vi "파일 I_O 실습.vi"() -> ()   [LabVIEW 2020]
uses:
  <vilib>/Utility/sysdir.llb/System Directory Type.ctl
  <vilib>/Utility/file.llb/Read Delimited Spreadsheet (DBL).vi
panel:
  out "연결된 문자열":string
  out "all rows":dbl[][](array[numeric]) caption="모든 행"
  out "데이터 2":string[][](array[string])
  out "데이터":dbl[](array[numeric])
  out "추가된 경로":path
  out "system directory":path caption="시스템 디렉토리"
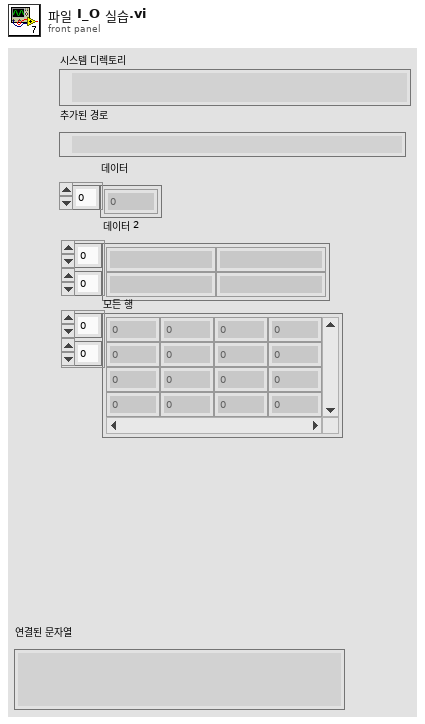
[diagram p1: front panel]
types:
  T1 = enum16{"open", "replace", "create", "open or create", "replace or create", "replace or create with confirmation"}
  T2 = typedef "System Directory Type.ctl" = i32
  T3 = enum16{"open", "open or create", "create or replace", "create", "open (read-only)"}
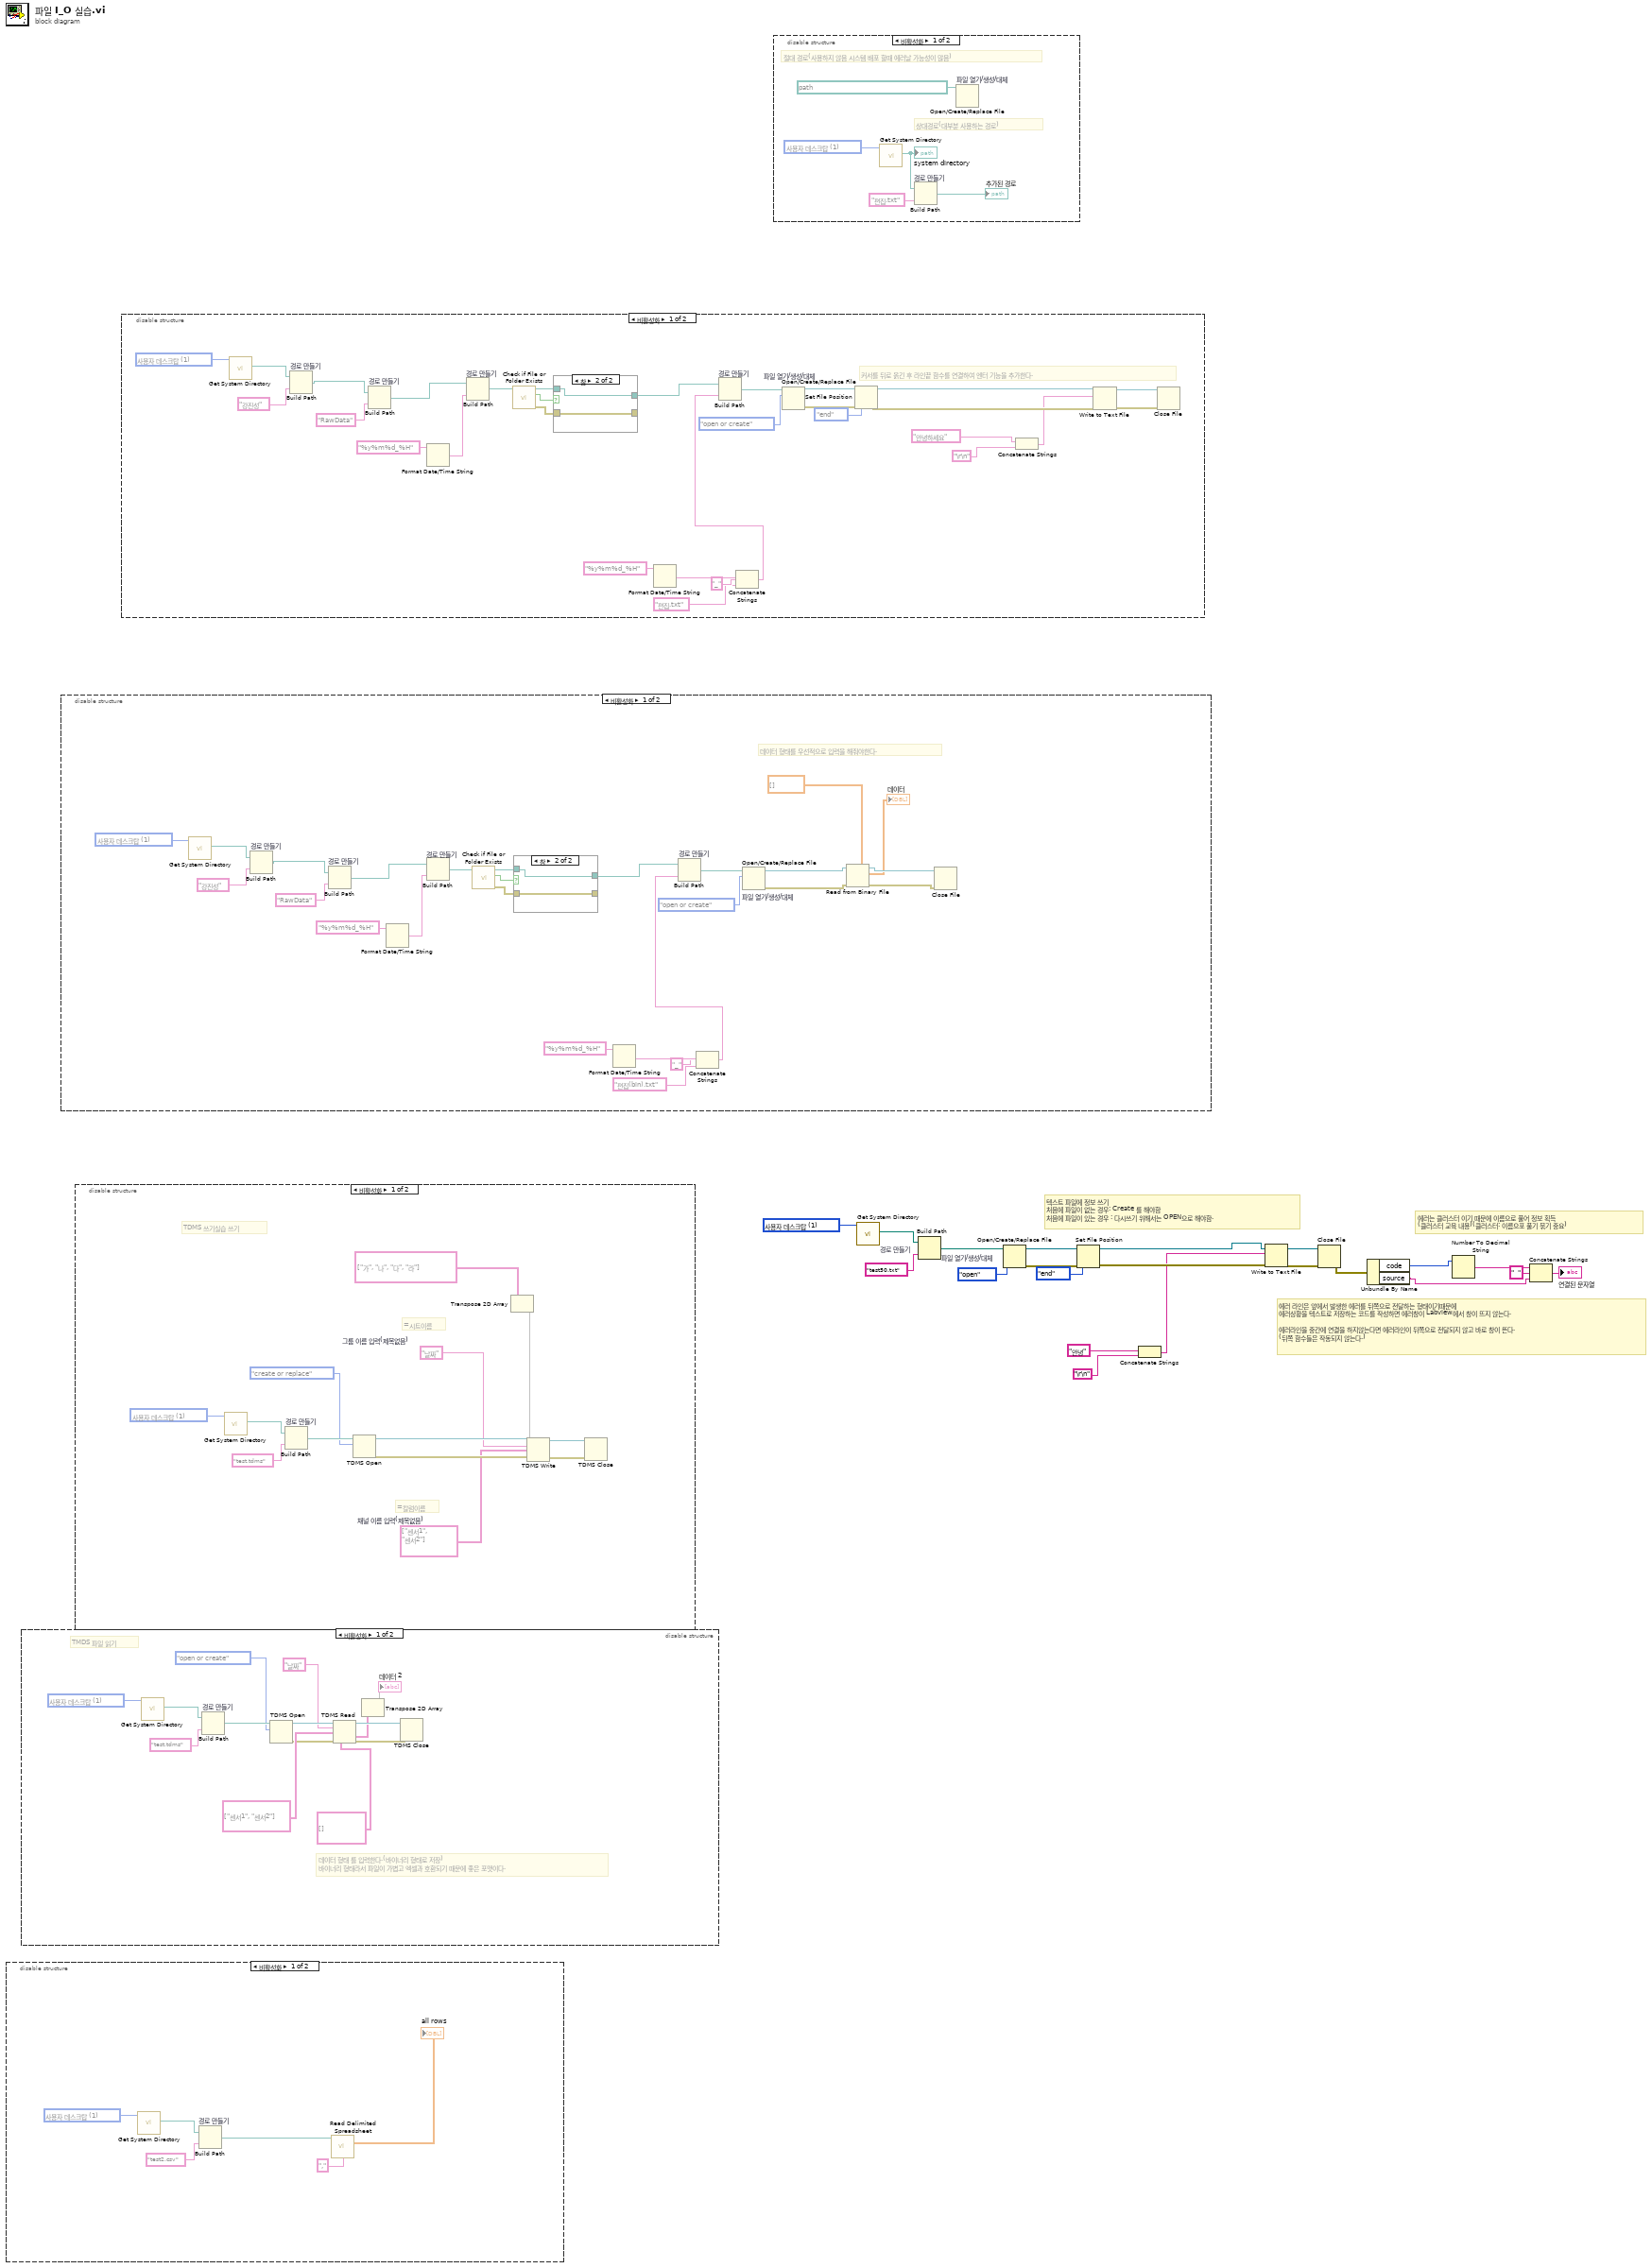
[diagram p0: block diagram]
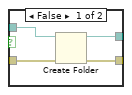
[diagram p5: hidden frame]
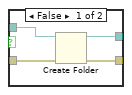
[diagram p7: hidden frame]
diagram:
  w21 = T2 1 items=["사용자 홈"=0, "사용자 데스크탑"=1, "사용자 문서"=2, "사용자 어플리케이션 데이터"=3, "사용자 환경"=4, "사용자 임시"=5, "퍼블릭 문서"=6, "퍼블릭 어플리케이션 데이터"=7, "퍼블릭 환경"=8, "퍼블릭 캐시"=13, "시스템 코어 라이브러리"=9, "시스템 설치된 라이브러리"=10, "어플리케이션 파일"=11, "부팅 볼륨 루트"=12] ("system directory type")
  # "에러 라인은 앞에서 발생한 에러를 뒤쪽으로 전달하는 형태이기때문에\n에러상황을 텍스트로 저장하는 코드를 작성하면 에러창이 Labview에서 창이 뜨지 않는다.\n\n에러라인을 중간에 연결을 하지않는다면 에러라인이 뒤쪽으로 전달되지 않고 바로 창이 뜬다.\n(뒤쪽 함수들은 작동되지 않는다.)"
  # "에러는 클러스터 이기 때문에 이름으로 풀어 정보 획득\n(클러스터 교육 내용)(클러스터: 이름으포 풀기 묶기 중요)"
  # "텍스트 파일에 정보 쓰기\n처음에 파일이 없는 경우: Create 를 해야함\n처음에 파일이 있는 경우 : 다시쓰기 위해서는 OPEN으로 해야함."
  n1 = disable-structure shown="비활성화" {
    frame Disabled {
      w27 = T2 1 items=["사용자 홈"=0, "사용자 데스크탑"=1, "사용자 문서"=2, "사용자 어플리케이션 데이터"=3, "사용자 환경"=4, "사용자 임시"=5, "퍼블릭 문서"=6, "퍼블릭 어플리케이션 데이터"=7, "퍼블릭 환경"=8, "퍼블릭 캐시"=13, "시스템 코어 라이브러리"=9, "시스템 설치된 라이브러리"=10, "어플리케이션 파일"=11, "부팅 볼륨 루트"=12] ("system directory type")
      n2 = call <vilib>:"Get System Directory.vi"("system directory type"=w27) -> ("system directory"=w26:path)  [unwired: 10 in]
      n3 = Build Path "경로 만들기"(base path=w26, name or relative path="test2.csv") -> (appended path=w24:path)
      n4 = call-poly <vilib>:"Read Delimited Spreadsheet.vi"("file path (dialog if empty)"=w24, "delimiter (\\t)"="," ("delimiter (\\t)")) -> ("all rows"=→"all rows":dbl[][])  [unwired: 8 in, 5 out]
    }
    frame Enabled {
    }
  }
  n5 = disable-structure shown="비활성화" {
    frame Disabled {
      w41 = T2 1 items=["사용자 홈"=0, "사용자 데스크탑"=1, "사용자 문서"=2, "사용자 어플리케이션 데이터"=3, "사용자 환경"=4, "사용자 임시"=5, "퍼블릭 문서"=6, "퍼블릭 어플리케이션 데이터"=7, "퍼블릭 환경"=8, "퍼블릭 캐시"=13, "시스템 코어 라이브러리"=9, "시스템 설치된 라이브러리"=10, "어플리케이션 파일"=11, "부팅 볼륨 루트"=12] ("system directory type")
      # "데이터 형태 를 입력한다.(바이너리 형태로 저장)\n바이너리 형태라서 파일이 가볍고 엑셀과 호환되기 때문에 좋은 포맷이다."
      # "TMDS 파일 읽기"
      n6 = call <vilib>:"Get System Directory.vi"("system directory type"=w41) -> ("system directory"=w40:path)  [unwired: 10 in]
      n7 = Build Path "경로 만들기"(base path=w40, name or relative path="test.tdms") -> (appended path=w38:path)
      n8 = TDMS Open(10:T3."open or create" ("동작(0:open)"), 11:w38) -> (0:w31:errorcluster, 3:w36:refnum<k34>)  [unwired: 5 in]
      n9 = TDMS Read(0:w36, 5:"날짜" ("그룹 이름 입력"), 7:string[] ["센서1", "센서2"] ("채널 이름 입력"), 11:w31, 12:string[][] []) -> (4:w33:refnum<k34>, 10:w29:string[][], 15:w32:errorcluster)  [unwired: 3 in, 3 out]
      n10 = Transpose 2D Array(2D array=w29) -> (transposed array=→"데이터 2":string[][])
      n11 = TDMS Close(8:w32, 11:w33) -> ()  [unwired: 2 out]
    }
    frame Enabled {
    }
  }
  n12 = disable-structure shown="비활성화" {
    frame Disabled {
      w67 = T2 1 items=["사용자 홈"=0, "사용자 데스크탑"=1, "사용자 문서"=2, "사용자 어플리케이션 데이터"=3, "사용자 환경"=4, "사용자 임시"=5, "퍼블릭 문서"=6, "퍼블릭 어플리케이션 데이터"=7, "퍼블릭 환경"=8, "퍼블릭 캐시"=13, "시스템 코어 라이브러리"=9, "시스템 설치된 라이브러리"=10, "어플리케이션 파일"=11, "부팅 볼륨 루트"=12] ("system directory type")
      # "데이터 형태를 우선적으로 입력을 해줘야한다."
      n13 = call <vilib>:"Get System Directory.vi"("system directory type"=w67) -> ("system directory"=w64:path)  [unwired: 10 in]
      n14 = Build Path "경로 만들기"(base path=w64, name or relative path="강진성") -> (appended path=w59:path)
      n15 = Build Path "경로 만들기"(base path=w59, name or relative path="RawData") -> (appended path=w58:path)
      n16 = Format Date/Time String(time format string (%c)="%y%m%d_%H" ("시간 포맷 문자열 (%c)")) -> (date/time string=w61:string)  [unwired: 2 in]
      n17 = Build Path "경로 만들기"(base path=w58, name or relative path=w61) -> (appended path=w52:path)
      n18 = call <vilib>:"Check if File or Folder Exists.vi"("path"=w52) -> ("error out"=w49:errorcluster, "file or folder exists?"=w51:bool, "dup path"=w50:path)  [unwired: 8 in]
      n19 = case shown="참" w51 {
        tunnel: w50 -> [w71 w73]
        tunnel: w49 -> [w70 w72]
        tunnel: [w69 w73] -> w48
        tunnel: [w68 w72] -> _
        frame False {
          n20 = Create Folder(path (use dialog)=w71, error in=w70) -> (created path=w69:path, error out=w68:errorcluster)  [unwired: 1 in, 1 out]
        }
        frame True {
        }
      }
      n21 = Format Date/Time String(time format string (%c)="%y%m%d_%H" ("시간 포맷 문자열 (%c)")) -> (date/time string=w56:string)  [unwired: 2 in]
      n22 = Concatenate Strings(w56, "_" ("문자열"), "편집(bin).txt") -> (w53:string)
      n23 = Build Path "경로 만들기"(base path=w48, name or relative path=w53) -> (appended path=w66:path)
      n24 = Open/Create/Replace File "파일 열기/생성/대체"(file path (use dialog)=w66, operation (0:open)=T1."open or create" ("동작(0:open)")) -> (refnum out=w47:refnum<file>, error out=w46:errorcluster)  [unwired: 4 in, 1 out]
      n25 = Read from Binary File(5:dbl[] [], 8:w46, 11:w47) -> (0:w44:errorcluster, 2:→"데이터":dbl[], 3:w45:refnum<file>)  [unwired: 3 in, 1 out]
      n26 = Close File(refnum=w45, error in=w44) -> ()  [unwired: 2 out]
    }
    frame Enabled {
    }
  }
  n27 = disable-structure shown="비활성화" {
    frame Disabled {
      w75 = string[] ["센서1", "센서2"]  # 채널 이름 입력(제목없음)
      w76 = "날짜"  # 그룹 이름 입력(제목없음)
      w86 = T2 1 items=["사용자 홈"=0, "사용자 데스크탑"=1, "사용자 문서"=2, "사용자 어플리케이션 데이터"=3, "사용자 환경"=4, "사용자 임시"=5, "퍼블릭 문서"=6, "퍼블릭 어플리케이션 데이터"=7, "퍼블릭 환경"=8, "퍼블릭 캐시"=13, "시스템 코어 라이브러리"=9, "시스템 설치된 라이브러리"=10, "어플리케이션 파일"=11, "부팅 볼륨 루트"=12] ("system directory type")
      # "TDMS 쓰기실습 쓰기"
      # "=칼럼이름"
      # "=시트이름"
      n28 = call <vilib>:"Get System Directory.vi"("system directory type"=w86) -> ("system directory"=w85:path)  [unwired: 10 in]
      n29 = Build Path "경로 만들기"(base path=w85, name or relative path="test.tdms") -> (appended path=w83:path)
      n30 = TDMS Open(10:T3."create or replace" ("동작(0:open)"), 11:w83) -> (0:w81:errorcluster, 3:w82:refnum<k34>)  [unwired: 5 in]
      n31 = Transpose 2D Array(2D array=string[][] [["가", "나"], ["다", "라"]]) -> (transposed array=w74:string[][])
      n32 = TDMS Write(0:w82, 5:w76, 7:w75, 9:w74, 11:w81) -> (4:w80:refnum<k34>, 15:w79:errorcluster)  [unwired: 1 in, 2 out]
      n33 = TDMS Close(8:w79, 11:w80) -> ()  [unwired: 2 out]
    }
    frame Enabled {
    }
  }
  n34 = disable-structure shown="비활성화" {
    frame Disabled {
      w116 = T2 1 items=["사용자 홈"=0, "사용자 데스크탑"=1, "사용자 문서"=2, "사용자 어플리케이션 데이터"=3, "사용자 환경"=4, "사용자 임시"=5, "퍼블릭 문서"=6, "퍼블릭 어플리케이션 데이터"=7, "퍼블릭 환경"=8, "퍼블릭 캐시"=13, "시스템 코어 라이브러리"=9, "시스템 설치된 라이브러리"=10, "어플리케이션 파일"=11, "부팅 볼륨 루트"=12] ("system directory type")
      # "커서를 뒤로 옭긴 후 라인끝 함수를 연결하여 엔터 기능을 추가한다."
      n35 = call <vilib>:"Get System Directory.vi"("system directory type"=w116) -> ("system directory"=w113:path)  [unwired: 10 in]
      n36 = Build Path "경로 만들기"(base path=w113, name or relative path="강진성") -> (appended path=w108:path)
      n37 = Build Path "경로 만들기"(base path=w108, name or relative path="RawData") -> (appended path=w107:path)
      n38 = Format Date/Time String(time format string (%c)="%y%m%d_%H" ("시간 포맷 문자열 (%c)")) -> (date/time string=w110:string)  [unwired: 2 in]
      n39 = Build Path "경로 만들기"(base path=w107, name or relative path=w110) -> (appended path=w101:path)
      n40 = call <vilib>:"Check if File or Folder Exists.vi"("path"=w101) -> ("error out"=w98:errorcluster, "file or folder exists?"=w100:bool, "dup path"=w99:path)  [unwired: 8 in]
      n41 = case shown="참" w100 {
        tunnel: w99 -> [w120 w122]
        tunnel: w98 -> [w119 w121]
        tunnel: [w118 w122] -> w97
        tunnel: [w117 w121] -> _
        frame False {
          n42 = Create Folder(path (use dialog)=w120, error in=w119) -> (created path=w118:path, error out=w117:errorcluster)  [unwired: 1 in, 1 out]
        }
        frame True {
        }
      }
      n43 = Format Date/Time String(time format string (%c)="%y%m%d_%H" ("시간 포맷 문자열 (%c)")) -> (date/time string=w105:string)  [unwired: 2 in]
      n44 = Concatenate Strings(w105, "_" ("문자열"), "편집.txt") -> (w102:string)
      n45 = Build Path "경로 만들기"(base path=w97, name or relative path=w102) -> (appended path=w115:path)
      n46 = Open/Create/Replace File "파일 열기/생성/대체"(file path (use dialog)=w115, operation (0:open)=T1."open or create" ("동작(0:open)")) -> (refnum out=w94:refnum<file>, error out=w93:errorcluster)  [unwired: 4 in, 1 out]
      n47 = Set File Position(refnum=w94, from (0:start)=enum16{"start", "end", "current"}."end" ("위치(0:start)"), error in=w93) -> (refnum out=w91:refnum<file>, error out=w90:errorcluster)  [unwired: 1 in]
      n48 = Concatenate Strings("안녕하세요" ("텍스트"), "\r\n") -> (w87:string)
      n49 = Write to Text File(file (use dialog)=w91, text=w87, error in=w90) -> (refnum out=w96:refnum<file>, error out=w95:errorcluster)  [unwired: 1 in, 1 out]
      n50 = Close File(refnum=w96, error in=w95) -> ()  [unwired: 2 out]
    }
    frame Enabled {
    }
  }
  n51 = disable-structure shown="비활성화" {
    frame Disabled {
      w126 = T2 1 items=["사용자 홈"=0, "사용자 데스크탑"=1, "사용자 문서"=2, "사용자 어플리케이션 데이터"=3, "사용자 환경"=4, "사용자 임시"=5, "퍼블릭 문서"=6, "퍼블릭 어플리케이션 데이터"=7, "퍼블릭 환경"=8, "퍼블릭 캐시"=13, "시스템 코어 라이브러리"=9, "시스템 설치된 라이브러리"=10, "어플리케이션 파일"=11, "부팅 볼륨 루트"=12] ("system directory type")
      # "상대경로(대부분 사용하는 경로)"
      # "절대 경로(사용하지 않음 시스템 배포 할때 에러날 가능성이 많음)"
      n52 = call <vilib>:"Get System Directory.vi"("system directory type"=w126) -> ("system directory"=w125:path)  [unwired: 10 in]
      "system directory" <- w125
      n53 = Build Path "경로 만들기"(base path=w125, name or relative path="편집.txt") -> (appended path=→"추가된 경로":path)
      n54 = Open/Create/Replace File "파일 열기/생성/대체"(file path (use dialog)=path "C:/Users/shkim/Desktop/편집.txt") -> ()  [unwired: 5 in, 3 out]
    }
    frame Enabled {
    }
  }
  n55 = call <vilib>:"Get System Directory.vi"("system directory type"=w21) -> ("system directory"=w20:path)  [unwired: 10 in]
  n56 = Build Path "경로 만들기"(base path=w20, name or relative path="test50.txt") -> (appended path=w18:path)
  n57 = Open/Create/Replace File "파일 열기/생성/대체"(file path (use dialog)=w18, operation (0:open)=T1."open" ("동작(0:open)")) -> (refnum out=w14:refnum<file>, error out=w13:errorcluster)  [unwired: 4 in, 1 out]
  n58 = Set File Position(refnum=w14, from (0:start)=enum16{"start", "end", "current"}."end" ("위치(0:start)"), error in=w13) -> (refnum out=w12:refnum<file>, error out=w11:errorcluster)  [unwired: 1 in]
  n59 = Concatenate Strings("안녕" ("텍스트"), "\r\n") -> (w7:string)
  n60 = Write to Text File(file (use dialog)=w12, text=w7, error in=w11) -> (refnum out=w17:refnum<file>, error out=w16:errorcluster)  [unwired: 1 in, 1 out]
  n61 = Close File(refnum=w17, error in=w16) -> (error out=w6:errorcluster)  [unwired: 1 out]
  n62 = Unbundle By Name(w6) -> ("code"=w5:i32, "source"=w2:string)
  n63 = Number To Decimal String(number=w5) -> (decimal integer string=w4:string)  [unwired: 1 in]
  n64 = Concatenate Strings(w4, "  " ("문자열"), w2) -> (→"연결된 문자열":string)
